vi "EventDetected.vi"(5 "Channel":i32, 6 "error in":errorcluster) -> (0 "error out":errorcluster, 4 "Event":bool)   [LabVIEW 2014]
doc: "Returns True if one or more events on the specified channel has been detected since the last time this VI was called.\n\n\nAn event must be configured before calling this VI."
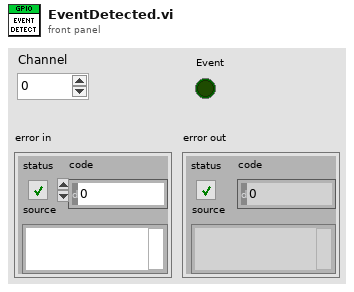
[diagram p1: front panel]
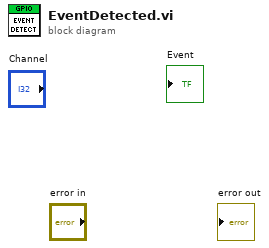
[diagram p0: block diagram]
diagram:
